vi "Inserisci acquisizione.vi"(6 "new element/subarray":string[](array[string]), 7 "Inserisci riga?":bool, 10 "indice prova":i32, 11 "Dati prove in 2":T1) -> (0 "Per tabella":string[][](array[string]), 1 "riga":string[](array[string]), 3 "Dati prove out 3":T1)   [LabVIEW 2019]
uses:
  TypeDef/Dati collaudo.ctl
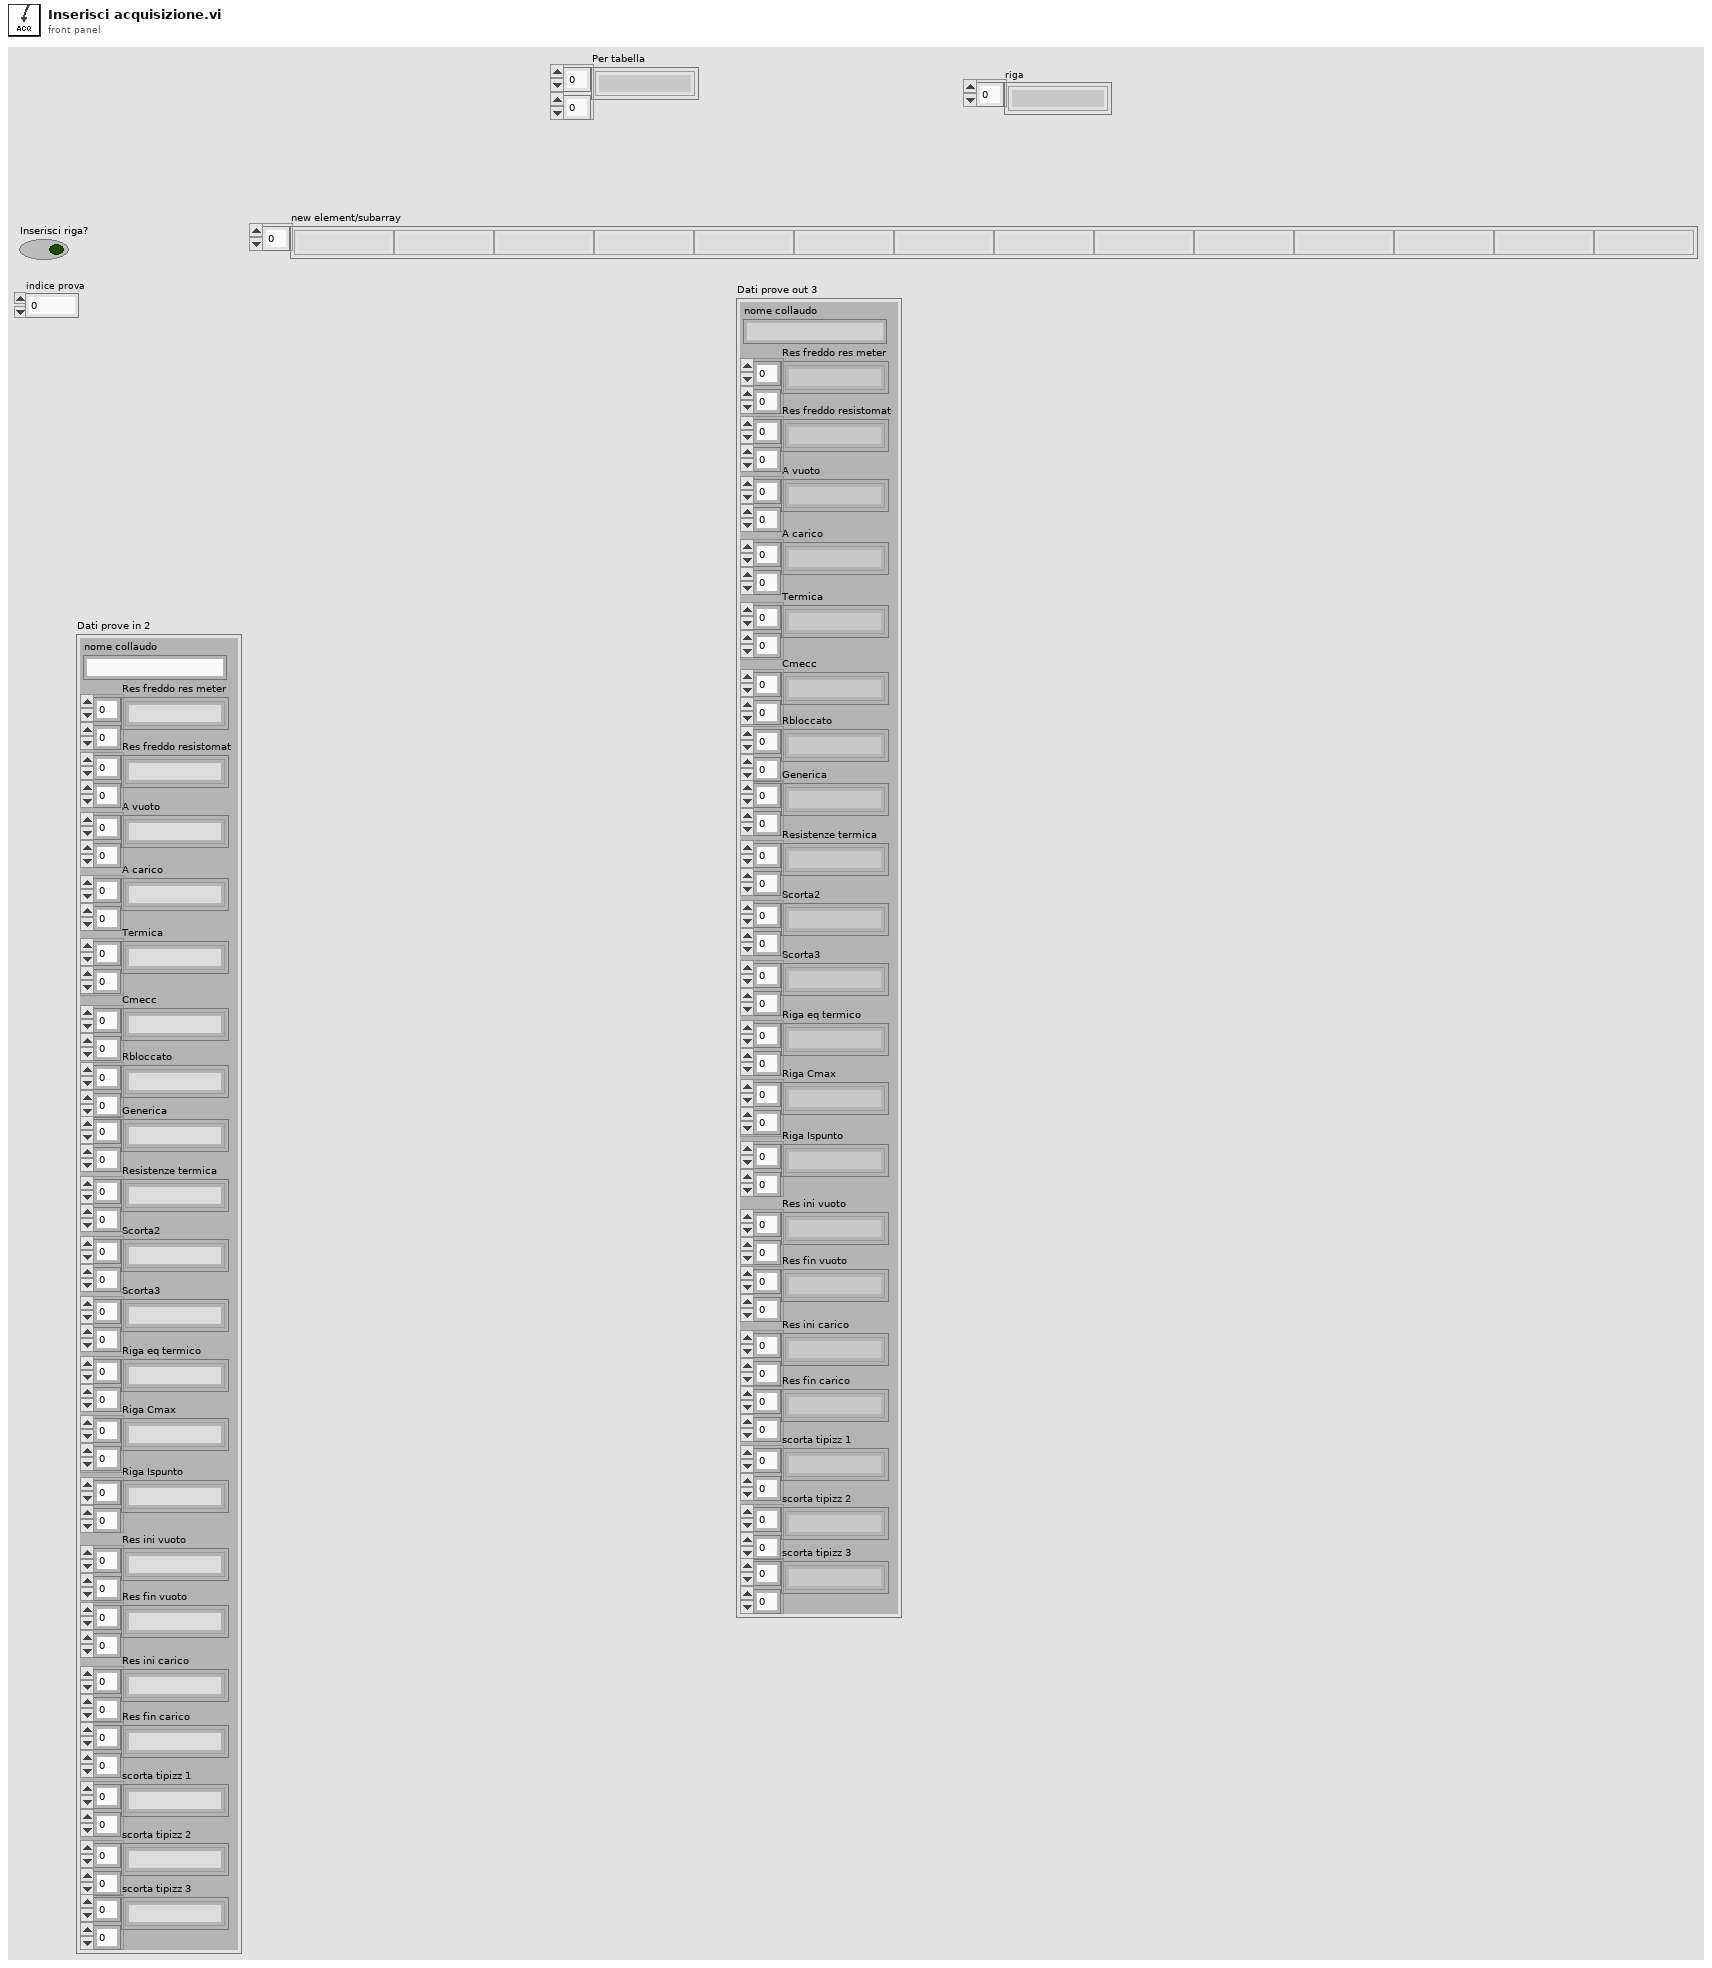
[diagram p1: front panel]
types:
  T1 = typedef "Dati collaudo.ctl" = cluster{"nome collaudo":string, "Res freddo res meter":string[][], "Res freddo resistomat":string[][], "A vuoto":string[][], "A carico":string[][], "Termica":string[][], "Cmecc":string[][], "Rbloccato":string[][], "Generica":string[][], "Resistenze termica":string[][], "Scorta2":string[][], "Scorta3":string[][], "Riga eq termico":string[][], "Riga Cmax":string[][], "Riga Ispunto":string[][], "Res ini vuoto":string[][], "Res fin vuoto":string[][], "Res ini carico":string[][], "Res fin carico":string[][], "scorta tipizz 1":string[][], "scorta tipizz 2":string[][], "scorta tipizz 3":string[][]}
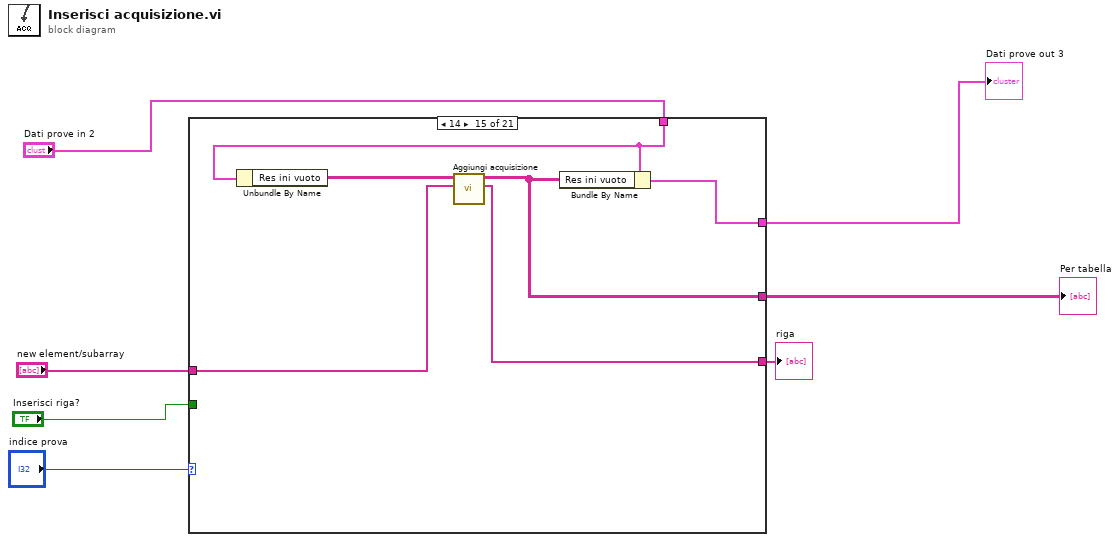
[diagram p0: block diagram]
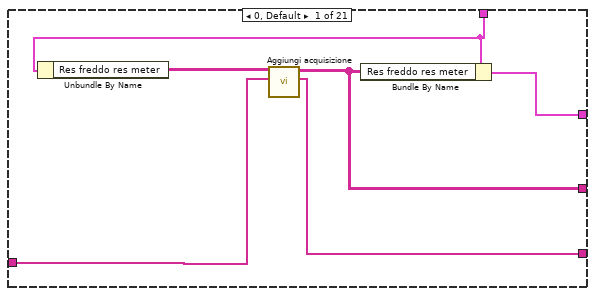
[diagram p2: hidden frame]
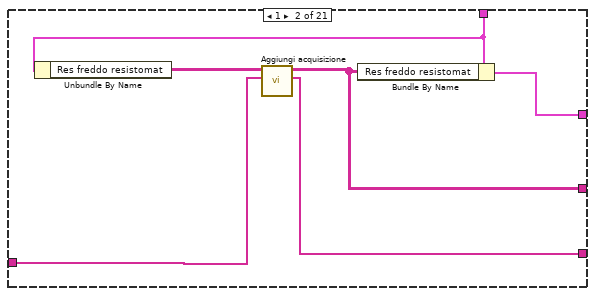
[diagram p3: hidden frame]
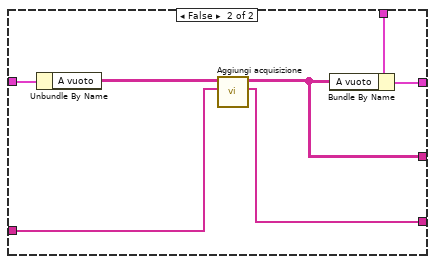
[diagram p5: hidden frame]
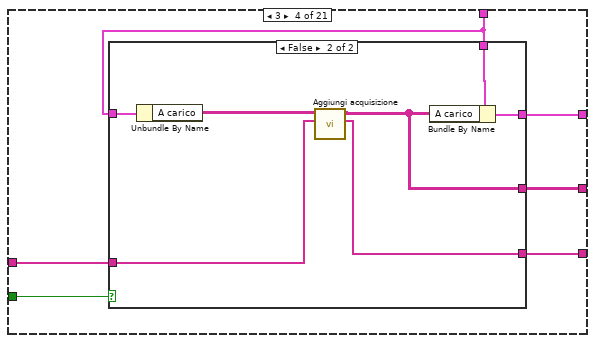
[diagram p6: hidden frame]
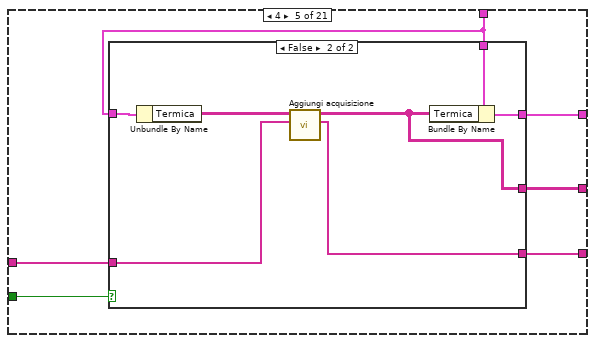
[diagram p8: hidden frame]
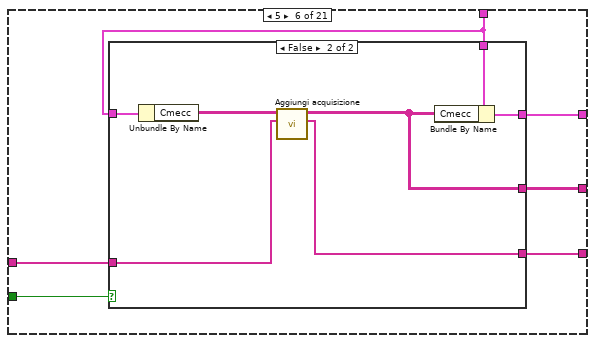
[diagram p10: hidden frame]
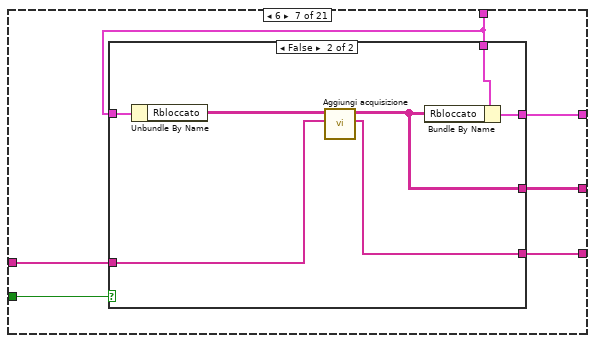
[diagram p12: hidden frame]
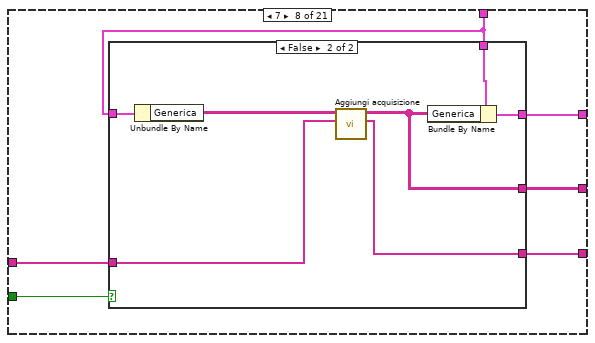
[diagram p14: hidden frame]
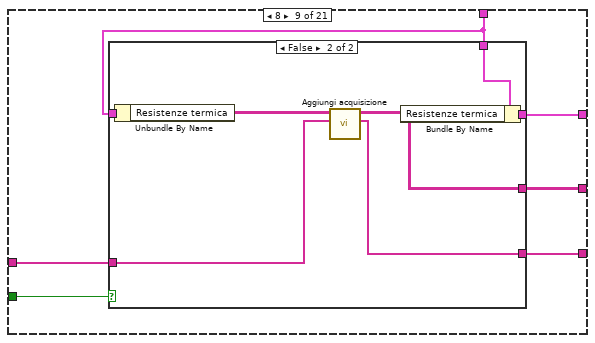
[diagram p16: hidden frame]
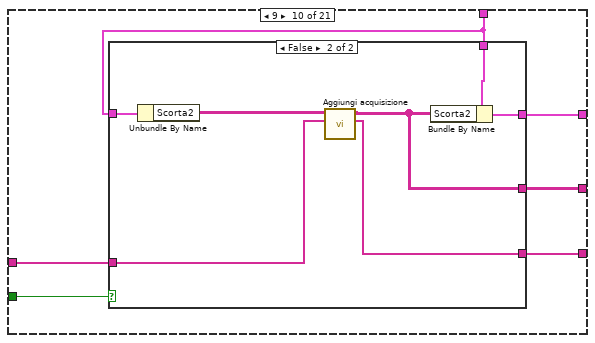
[diagram p18: hidden frame]
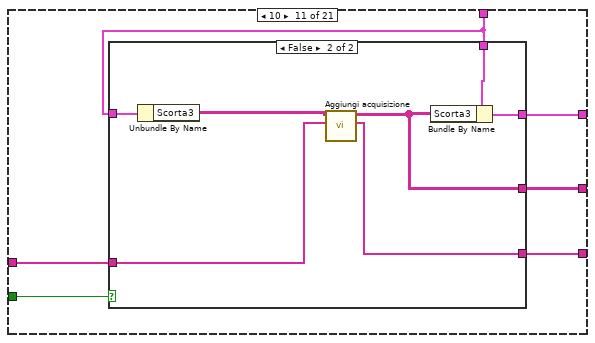
[diagram p20: hidden frame]
diagram:
  n1 = case shown="14" "indice prova" {
    tunnel: "new element/subarray" -> [w9 w15 w25 w39 w53 w67 w81 w95 w109 w123 w137 w147 w153 w159 w165 w171 w177 w183 w189 w195 w201]
    tunnel: "Inserisci riga?" -> [_ _ w24 w38 w52 w66 w80 w94 w108 w122 w136 _ _ _ _ _ _ _ _ _ _]
    tunnel: [w10 w16 w23 w37 w51 w65 w79 w93 w107 w121 w135 w148 w154 w160 w166 w172 w178 w184 w190 w196 w202] -> w5
    tunnel: [w13 w19 w22 w36 w50 w64 w78 w92 w106 w120 w134 w151 w157 w163 w169 w175 w181 w187 w193 w199 w205] -> w4
    tunnel: "Dati prove in 2" -> [w12 w18 w21 w35 w49 w63 w77 w91 w105 w119 w133 w150 w156 w162 w168 w174 w180 w186 w192 w198 w204]
    tunnel: [w8 w14 w20 w34 w48 w62 w76 w90 w104 w118 w132 w146 w152 w158 w164 w170 w176 w182 w188 w194 w200] -> w1
    frame 0, Default {
      n2 = Unbundle By Name(w12) -> ("Res freddo res meter"=w11:string[][])
      n3 = call "Aggiungi acquisizione.vi"("Nuova riga"=w9, "Dati in"=w11) -> ("riga"=w8:string[], "Dati out"=w10:string[][])  [unwired: 8 in]
      n4 = Bundle By Name(cluster=w12, "Res freddo res meter"=w10) -> (w13:T1)
    }
    frame 1 {
      n5 = Unbundle By Name(w18) -> ("Res freddo resistomat"=w17:string[][])
      n6 = call "Aggiungi acquisizione.vi"("Nuova riga"=w15, "Dati in"=w17) -> ("riga"=w14:string[], "Dati out"=w16:string[][])  [unwired: 8 in]
      n7 = Bundle By Name(cluster=w18, "Res freddo resistomat"=w16) -> (w19:T1)
    }
    frame 2 {
      n8 = case shown="True" w24 {
        tunnel: w25 -> [_ w28]
        tunnel: [_ w29] -> w23
        tunnel: [w26 w33] -> w22
        tunnel: w21 -> [w26 w32]
        tunnel: w21 -> [_ w31]
        tunnel: [_ w27] -> w20
        frame True {
        }
        frame False {
          n9 = Unbundle By Name(w31) -> ("A vuoto"=w30:string[][])
          n10 = call "Aggiungi acquisizione.vi"("Nuova riga"=w28, "Dati in"=w30) -> ("riga"=w27:string[], "Dati out"=w29:string[][])  [unwired: 8 in]
          n11 = Bundle By Name(cluster=w32, "A vuoto"=w29) -> (w33:T1)
        }
      }
    }
    frame 3 {
      n12 = case shown="False" w38 {
        tunnel: w39 -> [_ w42]
        tunnel: [_ w43] -> w37
        tunnel: [w40 w47] -> w36
        tunnel: w35 -> [w40 w46]
        tunnel: w35 -> [_ w45]
        tunnel: [_ w41] -> w34
        frame True {
        }
        frame False {
          n13 = Unbundle By Name(w45) -> ("A carico"=w44:string[][])
          n14 = call "Aggiungi acquisizione.vi"("Nuova riga"=w42, "Dati in"=w44) -> ("riga"=w41:string[], "Dati out"=w43:string[][])  [unwired: 8 in]
          n15 = Bundle By Name(cluster=w46, "A carico"=w43) -> (w47:T1)
        }
      }
    }
    frame 4 {
      n16 = case shown="False" w52 {
        tunnel: w53 -> [_ w57]
        tunnel: [_ w56] -> w51
        tunnel: [w54 w61] -> w50
        tunnel: w49 -> [w54 w60]
        tunnel: w49 -> [_ w59]
        tunnel: [_ w55] -> w48
        frame True {
        }
        frame False {
          n17 = Unbundle By Name(w59) -> ("Termica"=w58:string[][])
          n18 = call "Aggiungi acquisizione.vi"("Nuova riga"=w57, "Dati in"=w58) -> ("riga"=w55:string[], "Dati out"=w56:string[][])  [unwired: 8 in]
          n19 = Bundle By Name(cluster=w60, "Termica"=w56) -> (w61:T1)
        }
      }
    }
    frame 5 {
      n20 = case shown="False" w66 {
        tunnel: w67 -> [_ w71]
        tunnel: [_ w70] -> w65
        tunnel: [w68 w75] -> w64
        tunnel: w63 -> [w68 w74]
        tunnel: w63 -> [_ w73]
        tunnel: [_ w69] -> w62
        frame True {
        }
        frame False {
          n21 = Unbundle By Name(w73) -> ("Cmecc"=w72:string[][])
          n22 = call "Aggiungi acquisizione.vi"("Nuova riga"=w71, "Dati in"=w72) -> ("riga"=w69:string[], "Dati out"=w70:string[][])  [unwired: 8 in]
          n23 = Bundle By Name(cluster=w74, "Cmecc"=w70) -> (w75:T1)
        }
      }
    }
    frame 6 {
      n24 = case shown="False" w80 {
        tunnel: w81 -> [_ w84]
        tunnel: [_ w85] -> w79
        tunnel: [w82 w89] -> w78
        tunnel: w77 -> [w82 w88]
        tunnel: w77 -> [_ w87]
        tunnel: [_ w83] -> w76
        frame True {
        }
        frame False {
          n25 = Unbundle By Name(w87) -> ("Rbloccato"=w86:string[][])
          n26 = call "Aggiungi acquisizione.vi"("Nuova riga"=w84, "Dati in"=w86) -> ("riga"=w83:string[], "Dati out"=w85:string[][])  [unwired: 8 in]
          n27 = Bundle By Name(cluster=w88, "Rbloccato"=w85) -> (w89:T1)
        }
      }
    }
    frame 7 {
      n28 = case shown="False" w94 {
        tunnel: w95 -> [_ w98]
        tunnel: [_ w99] -> w93
        tunnel: [w96 w103] -> w92
        tunnel: w91 -> [w96 w102]
        tunnel: w91 -> [_ w101]
        tunnel: [_ w97] -> w90
        frame True {
        }
        frame False {
          n29 = Unbundle By Name(w101) -> ("Generica"=w100:string[][])
          n30 = call "Aggiungi acquisizione.vi"("Nuova riga"=w98, "Dati in"=w100) -> ("riga"=w97:string[], "Dati out"=w99:string[][])  [unwired: 8 in]
          n31 = Bundle By Name(cluster=w102, "Generica"=w99) -> (w103:T1)
        }
      }
    }
    frame 8 {
      n32 = case shown="False" w108 {
        tunnel: w109 -> [_ w112]
        tunnel: [_ w113] -> w107
        tunnel: [w110 w117] -> w106
        tunnel: w105 -> [w110 w116]
        tunnel: w105 -> [_ w115]
        tunnel: [_ w111] -> w104
        frame True {
        }
        frame False {
          n33 = Unbundle By Name(w115) -> ("Resistenze termica"=w114:string[][])
          n34 = call "Aggiungi acquisizione.vi"("Nuova riga"=w112, "Dati in"=w114) -> ("riga"=w111:string[], "Dati out"=w113:string[][])  [unwired: 8 in]
          n35 = Bundle By Name(cluster=w116, "Resistenze termica"=w113) -> (w117:T1)
        }
      }
    }
    frame 9 {
      n36 = case shown="False" w122 {
        tunnel: w123 -> [_ w126]
        tunnel: [_ w127] -> w121
        tunnel: [w124 w131] -> w120
        tunnel: w119 -> [w124 w130]
        tunnel: w119 -> [_ w129]
        tunnel: [_ w125] -> w118
        frame True {
        }
        frame False {
          n37 = Unbundle By Name(w129) -> ("Scorta2"=w128:string[][])
          n38 = call "Aggiungi acquisizione.vi"("Nuova riga"=w126, "Dati in"=w128) -> ("riga"=w125:string[], "Dati out"=w127:string[][])  [unwired: 8 in]
          n39 = Bundle By Name(cluster=w130, "Scorta2"=w127) -> (w131:T1)
        }
      }
    }
    frame 10 {
      n40 = case shown="False" w136 {
        tunnel: w137 -> [_ w140]
        tunnel: [_ w141] -> w135
        tunnel: [w138 w145] -> w134
        tunnel: w133 -> [w138 w144]
        tunnel: w133 -> [_ w143]
        tunnel: [_ w139] -> w132
        frame True {
        }
        frame False {
          n41 = Unbundle By Name(w143) -> ("Scorta3"=w142:string[][])
          n42 = call "Aggiungi acquisizione.vi"("Nuova riga"=w140, "Dati in"=w142) -> ("riga"=w139:string[], "Dati out"=w141:string[][])  [unwired: 8 in]
          n43 = Bundle By Name(cluster=w144, "Scorta3"=w141) -> (w145:T1)
        }
      }
    }
    frame 11 {
      n44 = Unbundle By Name(w150) -> ("Riga eq termico"=w149:string[][])
      n45 = call "Aggiungi acquisizione.vi"("Nuova riga"=w147, "Dati in"=w149) -> ("riga"=w146:string[], "Dati out"=w148:string[][])  [unwired: 8 in]
      n46 = Bundle By Name(cluster=w150, "Riga eq termico"=w148) -> (w151:T1)
    }
    frame 12 {
      n47 = Unbundle By Name(w156) -> ("Riga Cmax"=w155:string[][])
      n48 = call "Aggiungi acquisizione.vi"("Nuova riga"=w153, "Dati in"=w155) -> ("riga"=w152:string[], "Dati out"=w154:string[][])  [unwired: 8 in]
      n49 = Bundle By Name(cluster=w156, "Riga Cmax"=w154) -> (w157:T1)
    }
    frame 13 {
      n50 = Unbundle By Name(w162) -> ("Riga Ispunto"=w161:string[][])
      n51 = call "Aggiungi acquisizione.vi"("Nuova riga"=w159, "Dati in"=w161) -> ("riga"=w158:string[], "Dati out"=w160:string[][])  [unwired: 8 in]
      n52 = Bundle By Name(cluster=w162, "Riga Ispunto"=w160) -> (w163:T1)
    }
    frame 14 {
      n53 = Unbundle By Name(w168) -> ("Res ini vuoto"=w167:string[][])
      n54 = call "Aggiungi acquisizione.vi"("Nuova riga"=w165, "Dati in"=w167) -> ("riga"=w164:string[], "Dati out"=w166:string[][])  [unwired: 8 in]
      n55 = Bundle By Name(cluster=w168, "Res ini vuoto"=w166) -> (w169:T1)
    }
    frame 15 {
      n56 = Unbundle By Name(w174) -> ("Res fin vuoto"=w173:string[][])
      n57 = call "Aggiungi acquisizione.vi"("Nuova riga"=w171, "Dati in"=w173) -> ("riga"=w170:string[], "Dati out"=w172:string[][])  [unwired: 8 in]
      n58 = Bundle By Name(cluster=w174, "Res fin vuoto"=w172) -> (w175:T1)
    }
    frame 16 {
      n59 = Unbundle By Name(w180) -> ("Res ini carico"=w179:string[][])
      n60 = call "Aggiungi acquisizione.vi"("Nuova riga"=w177, "Dati in"=w179) -> ("riga"=w176:string[], "Dati out"=w178:string[][])  [unwired: 8 in]
      n61 = Bundle By Name(cluster=w180, "Res ini carico"=w178) -> (w181:T1)
    }
    frame 17 {
      n62 = Unbundle By Name(w186) -> ("Res fin carico"=w185:string[][])
      n63 = call "Aggiungi acquisizione.vi"("Nuova riga"=w183, "Dati in"=w185) -> ("riga"=w182:string[], "Dati out"=w184:string[][])  [unwired: 8 in]
      n64 = Bundle By Name(cluster=w186, "Res fin carico"=w184) -> (w187:T1)
    }
    frame 18 {
      n65 = Unbundle By Name(w192) -> ("scorta tipizz 1"=w191:string[][])
      n66 = call "Aggiungi acquisizione.vi"("Nuova riga"=w189, "Dati in"=w191) -> ("riga"=w188:string[], "Dati out"=w190:string[][])  [unwired: 8 in]
      n67 = Bundle By Name(cluster=w192, "scorta tipizz 1"=w190) -> (w193:T1)
    }
    frame 19 {
      n68 = Unbundle By Name(w198) -> ("scorta tipizz 2"=w197:string[][])
      n69 = call "Aggiungi acquisizione.vi"("Nuova riga"=w195, "Dati in"=w197) -> ("riga"=w194:string[], "Dati out"=w196:string[][])  [unwired: 8 in]
      n70 = Bundle By Name(cluster=w198, "scorta tipizz 2"=w196) -> (w199:T1)
    }
    frame 20 {
      n71 = Unbundle By Name(w204) -> ("scorta tipizz 3"=w203:string[][])
      n72 = call "Aggiungi acquisizione.vi"("Nuova riga"=w201, "Dati in"=w203) -> ("riga"=w200:string[], "Dati out"=w202:string[][])  [unwired: 8 in]
      n73 = Bundle By Name(cluster=w204, "scorta tipizz 3"=w202) -> (w205:T1)
    }
  }
  "Per tabella" <- w5
  "Dati prove out 3" <- w4
  "riga" <- w1
